vi "generate header file.vi"(8 "error in (no error)":errorcluster, 10 "file path":path, 11 "shared memory editor node in":refnum<class "module editor node.lvclass">) -> (0 "error out":errorcluster, 3 "shared memory editor node out":refnum<class "module editor node.lvclass">)   [LabVIEW 2013, in "Shared Memory editor node.lvclass"]
uses:
  Shared Memory editor node.lvclass
  <vilib>/NI/DCAF/Tag Editor Core/Configuration Editor/Classes/Module editor node/module editor node.lvclass
  cheddar/C Header Generator.lvlib
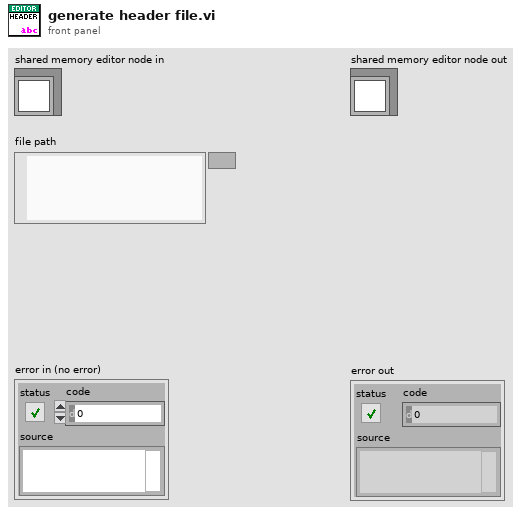
[diagram p1: front panel]
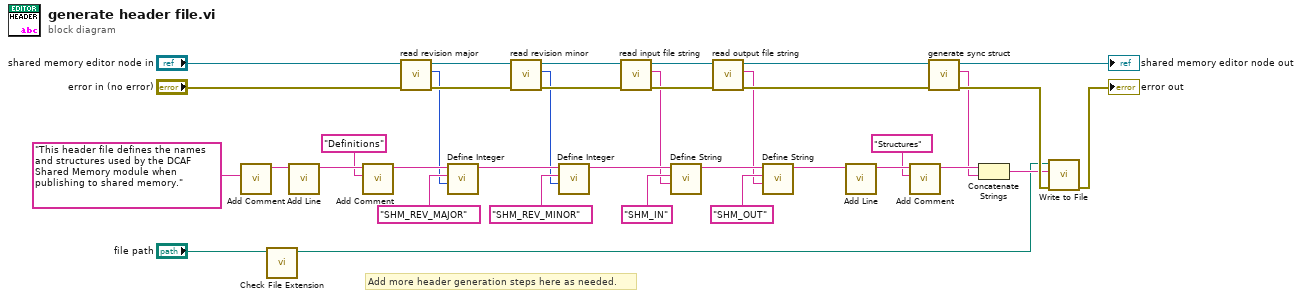
[diagram p0: block diagram]
diagram:
  # "Add more header generation steps here as needed."
  n1 = call "Add Comment.vi"("Comment"="This header file defines the names and structures used by the DCAF Shared Memory module when publishing to shared memory.") -> ("String out"=w31:string)  [unwired: 10 in]
  n2 = call "Check File Extension.vi"("path in"="file path") -> ("path out"=w15:path)  [unwired: 10 in]
  n3 = call "Add Line.vi"("String in"=w31) -> ("String out"=w30:string)  [unwired: 10 in]
  n4 = call "Add Comment.vi"("Comment"="Definitions", "String in"=w30) -> ("String out"=w8:string)  [unwired: 9 in]
  n5 = call "read revision major.vi"("error in"="error in (no error)", "shared memory editor node"="shared memory editor node in") -> ("error out"=w13:errorcluster, "revision major"=w2:u8, "shared memory editor node out"=w10:refnum<class "module editor node.lvclass">)  [unwired: 7 in]
  n6 = call "Define Integer.vi"("Value"=w2, "Name"="SHM_REV_MAJOR", "String in"=w8) -> ("String out"=w7:string)  [unwired: 8 in]
  n7 = call "read revision minor.vi"("error in"=w13, "shared memory editor node"=w10) -> ("error out"=w14:errorcluster, "revision minor"=w3:u8, "shared memory editor node out"=w11:refnum<class "module editor node.lvclass">)  [unwired: 7 in]
  n8 = call "Define Integer.vi"("Value"=w3, "Name"="SHM_REV_MINOR", "String in"=w7) -> ("String out"=w6:string)  [unwired: 8 in]
  n9 = call "read input file string.vi"("error in"=w14, "shared memory editor node"=w11) -> ("error out"=w23:errorcluster, "input file string"=w1:string, "shared memory editor node out"=w34:refnum<class "module editor node.lvclass">)  [unwired: 7 in]
  n10 = call "Define String.vi"("Value"=w1, "Name"="SHM_IN", "String in"=w6) -> ("String out"=w32:string)  [unwired: 8 in]
  n11 = call "read output file string.vi"("error in"=w23, "shared memory editor node"=w34) -> ("error out"=w22:errorcluster, "output file string"=w19:string, "shared memory editor node out"=w25:refnum<class "module editor node.lvclass">)  [unwired: 7 in]
  n12 = call "Define String.vi"("Value"=w19, "Name"="SHM_OUT", "String in"=w32) -> ("String out"=w28:string)  [unwired: 8 in]
  n13 = call "Add Line.vi"("String in"=w28) -> ("String out"=w27:string)  [unwired: 10 in]
  n14 = call "Add Comment.vi"("Comment"="Structures", "String in"=w27) -> ("String out"=w24:string)  [unwired: 9 in]
  n15 = call "generate sync struct.vi"("error in (no error)"=w22, "shared memory editor node in"=w25) -> ("error out"=w37:errorcluster, "struct string"=w20:string, "shared memory editor node out"=→"shared memory editor node out":refnum<class "module editor node.lvclass">)  [unwired: 7 in]
  n16 = Concatenate Strings(w24, w20) -> (w18:string)
  n17 = call "Write to File.vi"("error in (no error)"=w37, "header text"=w18, "file path"=w15) -> ("error out"=→"error out":errorcluster)  [unwired: 8 in]
